vi "Queue Message.vi"(8 "error in (no error)":errorcluster, 11 "Message":T1) -> (0 "error out":errorcluster)   [LabVIEW 2019]
uses:
  Comms/State Controller/Controls/Comms Loop States.ctl
  Typedefs/Sensor Types.ctl
  Typedefs/Message Types.ctl
  Typedefs/Message.ctl
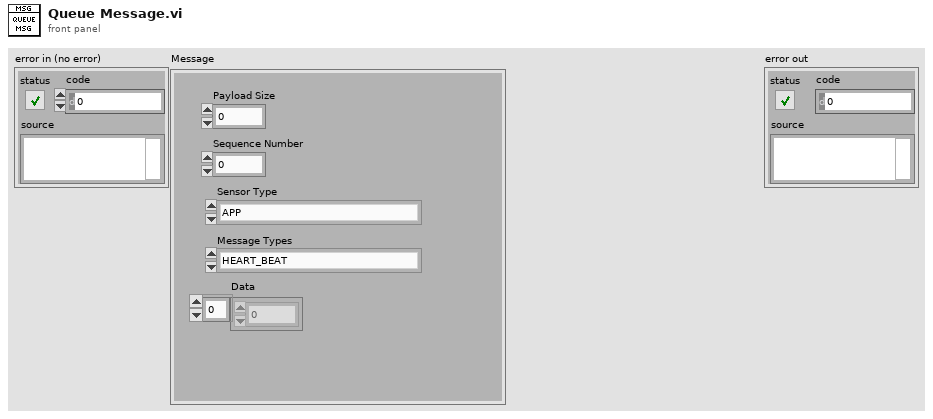
[diagram p1: front panel]
types:
  T1 = typedef "Message.ctl" = cluster{"Payload Size":u8, "Sequence Number":u8, "Sensor Type":T2, "Message Types":T3, "Data":u8[]}
  T2 = typedef "Sensor Types.ctl" = enum16{"APP", "TURBIDITY", "PH"}
  T3 = typedef "Message Types.ctl" = enum16{"HEART_BEAT", "CONNECT", "GET_CURRENT_MEASUREMENTS", "GET_LOG_FILE", "SEND_LOG_FILE_SIZE", "SEND_LOG_FILE_CHUNK", "GET_LOGGING_PERIOD", "SET_LOGGING_PERIOD", "SEND_SD_CARD_INFO", "GET_LOGS_LIST", "SEND_LOG_FILE_NAME", "SEND_LOGGING_PERIOD", "GET_RTC_TIME", "SET_RTC_TIME", "SEND_RTC_TIME", "SEND_CURRENT_MEASUREMENTS", "DELETE_LOG_FILE", "GET_SD_CARD_INFO", "GET_BATTERY_INFO", "SEND_BATTERY_INFO", "GET_LOG_FILE_SIZE", "ERROR_MSG"}
  T4 = typedef "Comms Loop States.ctl" = enum16{"Initalise", "User Event", "HEART_BEAT", "SEND_LOG_FILE_NAME", "Clear Log File Names", "SEND_LOG_FILE_CHUNK", "SEND_LOG_FILE_SIZE", "SEND_SD_CARD_INFO", "SEND_BATTERY_INFO", "SEND_LOGGING_PERIOD", "SEND_RTC_TIME", "SEND_CURRENT_MEASUREMENTS", "ERROR_MSG", "Clear Error Messages", "Send Message"}
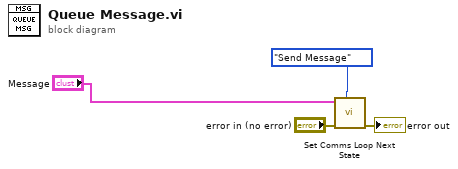
[diagram p0: block diagram]
diagram:
  n1 = call "Set Comms Loop Next State.vi"("Command"=Comms_Loop_States."Send Message", "error in (no error)"="error in (no error)", "Data"="Message") -> ("error out"=→"error out":errorcluster)  [unwired: 8 in]
